vi "PXI-Find 1st 16-bit Board.vi"(8 "error in (no error)":errorcluster) -> (0 "error out":errorcluster, 1 "Is M-series board":bool, 2 "DAQmx Device Name":tag)   [LabVIEW 2020]
uses:
  <resource>/objmgr/daqmx.rc
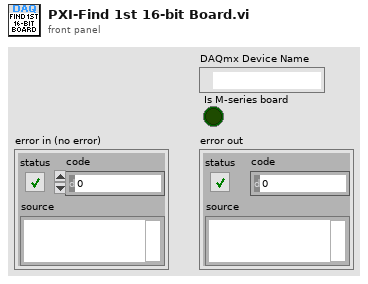
[diagram p1: front panel]
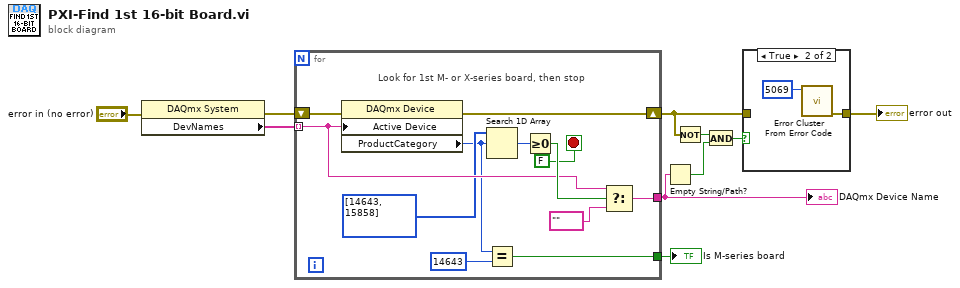
[diagram p0: block diagram]
diagram:
  n1 = property class="DAQmx System"(error in="error in (no error)") -> (error out=w9:errorcluster, "DevNames"=w8:tag[])  [unwired: 1 in, 1 out]
  n2 = for {
    tunnel: w8 -> [w19] mode=indexing
    shift-right: [w21] -> w2
    shift-left: w9 -> [w22]
    tunnel: [w17] -> w10
    tunnel: [w12] -> w1
    stop <- FALSE stop-if-true
    # "Look for 1st M- or X-series board, then stop"
    n3 = property class="DAQmx Device"(error in=w22, "Active Device"=w19) -> (error out=w21:errorcluster, "ProductCategory"=w14:i32)  [unwired: 1 in, 1 out]
    n4 = Search 1D Array(1D array=i32[] [14643, 15858], element=w14) -> (index of element=w15:i32)  [unwired: 1 in]
    n5 = Equal?(x=w14, y=14643) -> (x = y?=w12:bool)
    n6 = Greater Or Equal To 0?(x=w15) -> (x >= 0?=w20:bool)
    n7 = Select(t=w19, s=w20, f=tag "") -> (s? t:f=w17:tag)
  }
  "DAQmx Device Name" <- w10
  "Is M-series board" <- w1
  n8 = Empty String/Path?(string/path=w10) -> (empty?=w5:bool)
  n9 = Not(x=w2) -> (.not. x?=w3:bool)
  n10 = And(x=w3, y=w5) -> (x .and. y?=w6:bool)
  n11 = case shown="True" w6 {
    tunnel: [w23 w25] -> w4
    tunnel: w2 -> [w23 _]
    frame False {
    }
    frame True {
      n12 = call <vilib>:"Error Cluster From Error Code.vi"("error code (0)"=5069) -> ("error out"=w25:errorcluster)  [unwired: 8 in]
    }
  }
  "error out" <- w4
